vi "TwGetSpecXaxisFromShMem.vi"(3 "Axis type":i32, 4 "SpecAxis in":dbl[](array[numeric]), 5 "error in (no error)":errorcluster) -> (0 "UnitLabel":string, 1 "SpecAxis out":dbl[](array[numeric]), 2 "error out":errorcluster)   [LabVIEW 2009]
uses:
  TofDaqDll.dll
panel:
  in  "MaxMass":dbl
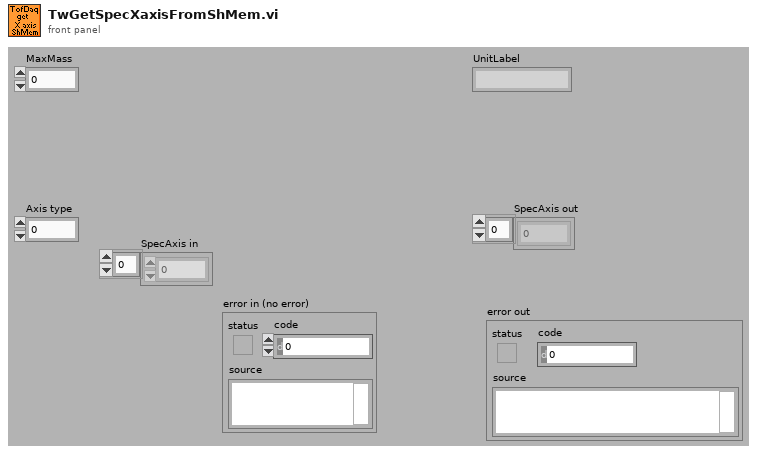
[diagram p1: front panel]
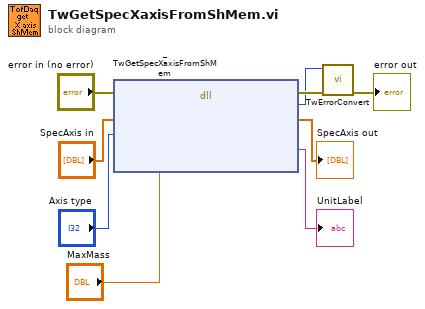
[diagram p0: block diagram]
diagram:
  n1 = dll-call lib="C:/Users/TofEmp/Desktop/LVTest/TofDaqDll.dll" fn="_TwGetSpecXaxisFromShMem"(error in="error in (no error)", "SpecAxis"="SpecAxis in", "Type"="Axis type", "MaxMass"="MaxMass") -> (error out=w8:errorcluster, "TwRetVal"=w7:i32, "SpecAxis"=→"SpecAxis out":dbl[], "UnitLabel"=→"UnitLabel":string)  [unwired: 4 in, 2 out]
  n2 = call "TwErrorConvert.vi"("error in (no error)"=w8, "error code"=w7) -> ("error out"=→"error out":errorcluster)  [unwired: 9 out]
